vi "TestFramework.vi"(8 "error in (no error)":errorcluster, 9 "Simulate Error?":bool) -> (0 "error out":errorcluster, 3 "Pass?":bool)   [LabVIEW 2017]
uses:
  builds/Data Sharing Framework/Current/Data Sharing Framework Core/DSF Core.lvlibp/Configuration/Public/Controls/DSF Engine Transfer Group Configuration.ctl
  builds/Data Sharing Framework/Current/Data Sharing Framework Core/DSF Core.lvlibp/Configuration/Public/Controls/DSF Direction.ctl
  builds/Data Sharing Framework/Current/Data Sharing Framework Core/DSF Core.lvlibp/Configuration/Public/Controls/DSF Timing Info.ctl
  builds/Data Sharing Framework/Current/Data Sharing Framework Core/DSF Core.lvlibp/Configuration/Public/Controls/DSF Engine Transfer Configuration.ctl
  builds/Data Sharing Framework/Current/Data Sharing Framework Core/DSF Core.lvlibp/Configuration/Public/Controls/DSF Byte Order.ctl
  builds/Data Sharing Framework/Current/Data Sharing Framework Core/DSF Core.lvlibp/Configuration/Public/Controls/DSF Engine Channel Configuration.ctl
  builds/Data Sharing Framework/Current/Data Sharing Framework Core/DSF Core.lvlibp/Configuration/Public/Controls/DSF Data Type.ctl
  builds/Data Sharing Framework/Current/Data Sharing Framework Core/DSF Core.lvlibp/Configuration/Public/Controls/DSF Settings Info.ctl
  builds/Data Sharing Framework/Current/Data Sharing Framework Core/DSF Core.lvlibp/Engine/Classes/Transfer Group/Transfer Group.lvclass
  DSFPlugin Transceiver.lvclass
  builds/Data Sharing Framework/Current/Data Sharing Framework Core/DSF Core.lvlibp/Engine/Classes/Transceiver/Transceiver.lvclass
  <vilib>/ErrorRing/Error Ring.xnode
  builds/Data Sharing Framework/Current/Data Sharing Framework Core/DSF Core.lvlibp
panel:
  in  "Transfer Group in":refnum<class "Transfer Group.lvclass">
  in  "Transfer Groups Configurations":T1[](array[typedef])=[{"name"="Transmitter", "direction"=enum."Tx", "cycle timing"={"priority"=0, "decimation"=1, "offset"=0}, "Transfers"=[{"name"="Transfer", "byte order"=enum."big-endian", "channel configurations"=[{"engine offset"=0, "name"="Data", "data type"=enum."DBL", "count"=1, "buffer offset"=0}], "settings"=[]}], "settings"=[]}, {"name"="Receiver", "direction"=enum."Rx", "cycle timing"={"priority"=0, "decimation"=1, "offset"=0}, "Transfers"=[{"name"="Transfer", "byte order"=enum."big-endian", "channel configurations"=[{"engine offset"=0, "name"="Data", "data type"=enum."DBL", "count"=1, "buffer offset"=0}], "settings"=[]}], "settings"=[]}] {"Transfers"."channel configurations"."buffer offset" format="%d bytes"}
  out "class":string
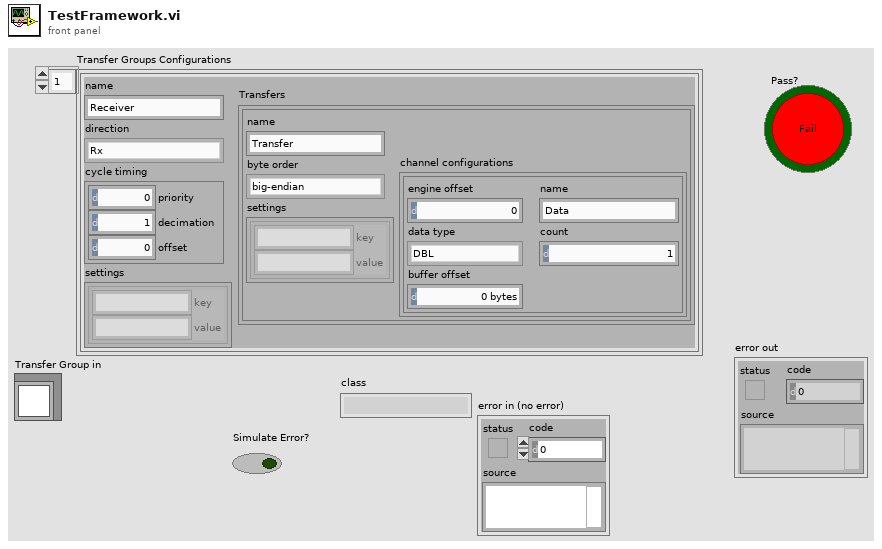
[diagram p1: front panel]
types:
  T1 = typedef "DSF Core.lvlibp/DSF Engine Transfer Group Configuration.ctl" = cluster{"name":string, "direction":T2, "cycle timing":T3, "Transfers":T4[], "settings":T8}
  T2 = typedef "DSF Core.lvlibp/DSF Direction.ctl" = enum8{"Tx", "Rx"}
  T3 = typedef "DSF Core.lvlibp/DSF Timing Info.ctl" = cluster{"priority":u64, "decimation":u64, "offset":u64}
  T4 = typedef "DSF Core.lvlibp/DSF Engine Transfer Configuration.ctl" = cluster{"name":string, "byte order":T5, "channel configurations":T6[], "settings":T8}
  T5 = typedef "DSF Core.lvlibp/DSF Byte Order.ctl" = enum8{"big-endian", "little-endian"}
  T6 = typedef "DSF Core.lvlibp/DSF Engine Channel Configuration.ctl" = cluster{"engine offset":u64, "name":string, "data type":T7, "count":u64, "buffer offset":u64}
  T7 = typedef "DSF Core.lvlibp/DSF Data Type.ctl" = enum8{"Bool", "SGL", "DBL", "I8", "I16", "I32", "I64", "U8", "U16", "U32", "U64"}
  T8 = typedef "DSF Core.lvlibp/DSF Settings Info.ctl" = cluster{"key":string, "value":string}[]
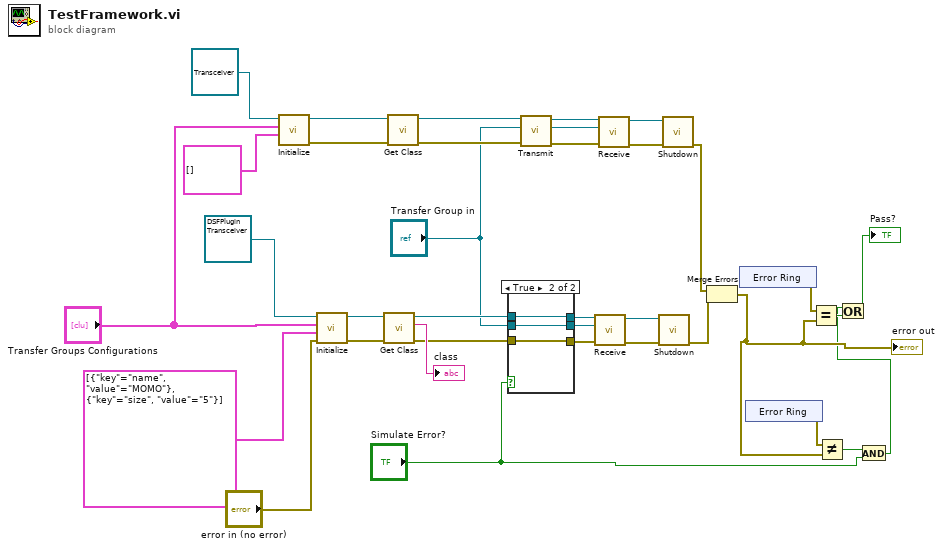
[diagram p0: block diagram]
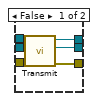
[diagram p2: hidden frame]
diagram:
  n1 = call-dynamic "Initialize.vi"("transceiver settings"=T8 [], "Transfer Groups Configurations"="Transfer Groups Configurations", "Transceiver in"=refnum<class "Transceiver.lvclass"> refnum) -> ("error out"=w14:errorcluster, "Transceiver out"=w15:refnum<class "Transceiver.lvclass">)  [unwired: 7 in]
  n2 = call-dynamic "Initialize.vi"("error in (no error)"="error in (no error)", "transceiver settings"=T8 [{"key"="name", "value"="MOMO"}, {"key"="size", "value"="5"}], "Transfer Groups Configurations"="Transfer Groups Configurations", "DSFPlugin in"=refnum<class "DSFPlugin Transceiver.lvclass"> refnum) -> ("error out"=w35:errorcluster, "DSFPlugin out"=w36:refnum<class "DSFPlugin Transceiver.lvclass">)  [unwired: 6 in]
  n3 = call-dynamic "Get Class.vi"("error in (no error)"=w35, "DSFPlugin Transceiver in"=w36) -> ("error out"=w31:errorcluster, "class"=→"class":string, "DSFPlugin Transceiver out"=w30:refnum<class "DSFPlugin Transceiver.lvclass">)  [unwired: 7 in]
  n4 = call-dynamic "Get Class.vi"("error in (no error)"=w14, "Transceiver in"=w15) -> ("error out"=w16:errorcluster, "Transceiver out"=w17:refnum<class "Transceiver.lvclass">)  [unwired: 7 in, 1 out]
  n5 = case shown="True" "Simulate Error?" {
    tunnel: w31 -> [w42 w44]
    tunnel: w30 -> [w41 w45]
    tunnel: [w40 w44] -> w29
    tunnel: [w39 w45] -> w28
    tunnel: [w38 w43] -> w25
    tunnel: "Transfer Group in" -> [w37 w43]
    frame False {
      n6 = call-dynamic "Transmit.vi"("error in (no error)"=w42, "Transfer Group in"=w37, "DSFPlugin in"=w41) -> ("error out"=w40:errorcluster, "Transfer Group out"=w38:refnum<class "Transfer Group.lvclass">, "DSFPlugin out"=w39:refnum<class "DSFPlugin Transceiver.lvclass">)  [unwired: 6 in]
    }
    frame True {
    }
  }
  n7 = call-dynamic "Transmit.vi"("error in (no error)"=w16, "Transfer Group in"="Transfer Group in", "Transceiver in"=w17) -> ("error out"=w18:errorcluster, "Transfer Group out"=w22:refnum<class "Transfer Group.lvclass">, "Transceiver out"=w19:refnum<class "Transceiver.lvclass">)  [unwired: 6 in]
  n8 = call-dynamic "Receive.vi"("error in (no error)"=w29, "Transfer Group in"=w25, "DSFPlugin in"=w28) -> ("error out"=w27:errorcluster, "DSFPlugin out"=w26:refnum<class "DSFPlugin Transceiver.lvclass">)  [unwired: 6 in, 1 out]
  n9 = call-dynamic "Receive.vi"("error in (no error)"=w18, "Transfer Group in"=w22, "Transceiver in"=w19) -> ("error out"=w20:errorcluster, "Transceiver out"=w21:refnum<class "Transceiver.lvclass">)  [unwired: 6 in, 1 out]
  n10 = call-dynamic "Shutdown.vi"("error in (no error)"=w27, "DSFPlugin in"=w26) -> ("error out"=w9:errorcluster)  [unwired: 8 in, 1 out]
  n11 = call-dynamic "Shutdown.vi"("error in (no error)"=w20, "Transceiver in"=w21) -> ("error out"=w8:errorcluster)  [unwired: 8 in, 1 out]
  n12 = Merge Errors(w8, w9) -> (w4:errorcluster)
  "error out" <- w4
  n13 = xnode "Error Ring"() -> ("error out"=w24:errorcluster)
  n14 = xnode "Error Ring"() -> ("error out"=w5:errorcluster)
  n15 = Equal?(x=w24, y=w4) -> (x = y?=w23:bool)
  n16 = Not Equal?(x=w5, y=w4) -> (x != y?=w3:bool)
  n17 = And(x=w3, y="Simulate Error?") -> (x .and. y?=w1:bool)
  n18 = Or(x=w1, y=w23) -> (x .or. y?=→"Pass?":bool)
